vi "pwm.vi"() -> ()   [LabVIEW 2021]
panel:
  out "Waveform Chart":dbl(graph)
  out "Boolean":bool
  in  "FREQ":dbl
  in  "DUTY":dbl(knob) scale=0.0..100.0
  in  "stop":bool
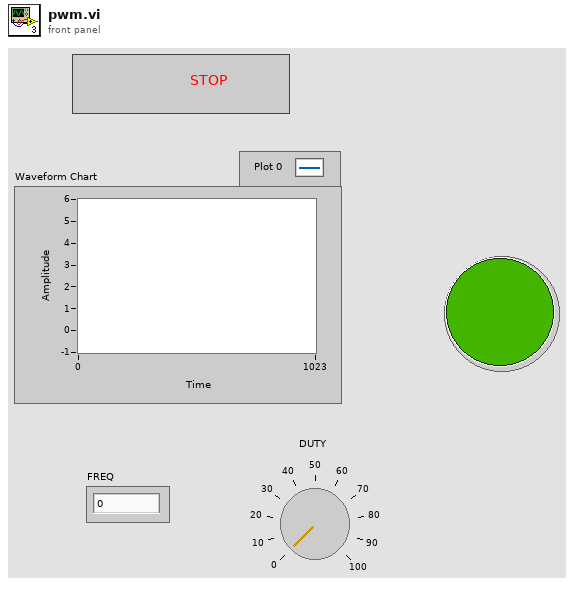
[diagram p1: front panel]
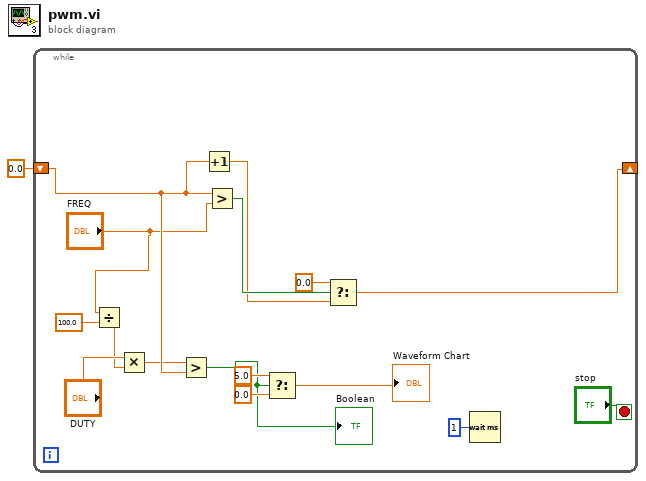
[diagram p0: block diagram]
diagram:
  n1 = while {
    shift-right: [w13] -> _
    shift-left: 0.0 -> [w10]
    stop <- "stop" stop-if-true
    n2 = Divide(x="FREQ", y=100.0) -> (x/y=w3:dbl)
    n3 = Multiply(x="DUTY", y=w3) -> (x*y=w7:dbl)
    n4 = Greater?(x=w7, y=w10) -> (0:w5:bool)
    "Boolean" <- w5
    n5 = Increment(x=w10) -> (x+1=w14:dbl)
    n6 = Greater?(x=w10, y="FREQ") -> (0:w16:bool)
    n7 = Select(t=5.0, s=w5, f=0.0) -> (s? t:f=→"Waveform Chart":dbl)
    n8 = Select(t=0.0, s=w16, f=w14) -> (s? t:f=w13:dbl)
    n9 = Wait (ms)(milliseconds to wait=u32 1) -> ()  [unwired: 1 out]
  }
